vi "Get NART response from response string.vi"(0 "Expected Response":T1, 5 "Response Subtype":T2, 7 "Expected Message start (\"\":any)":string, 9 "TCP Line":string, 11 "error in (no error)":errorcluster) -> (8 "NART Message":T3, 15 "error out":errorcluster)   [LabVIEW 2011, in "ART2 Test Panel.lvlib"]
uses:
  ART2 Test Panel.lvlib
  NART/Controls/NART Message.ctl
  NART/Controls/NART TCP Response Types.ctl
  NART/Controls/NART Response Subtype.ctl
  <vilib>/Utility/error.llb/whitespace.ctl
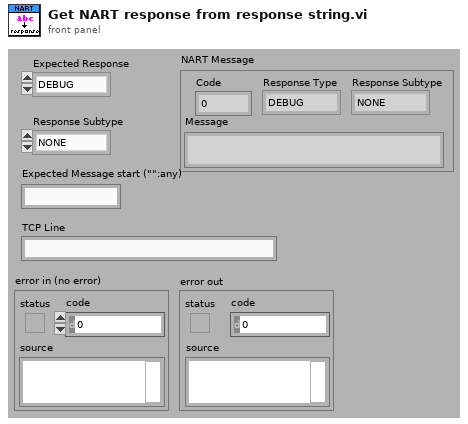
[diagram p1: front panel]
types:
  T1 = typedef "ART2 Test Panel.lvlib/NART TCP Response Types.ctl" = enum16{"DEBUG", "CONTROL", "INFO", "WARNING", "ERROR", "NONE"}
  T2 = typedef "ART2 Test Panel.lvlib/NART Response Subtype.ctl" = enum16{"NONE", "OK", "ON", "OFF", "BEGIN", "DONE"}
  T3 = typedef "ART2 Test Panel.lvlib/NART Message.ctl" = cluster{"Code":dbl, "Response Type":T1, "Response Subtype":T2, "Message":string}
  T4 = typedef "whitespace.ctl" = u16
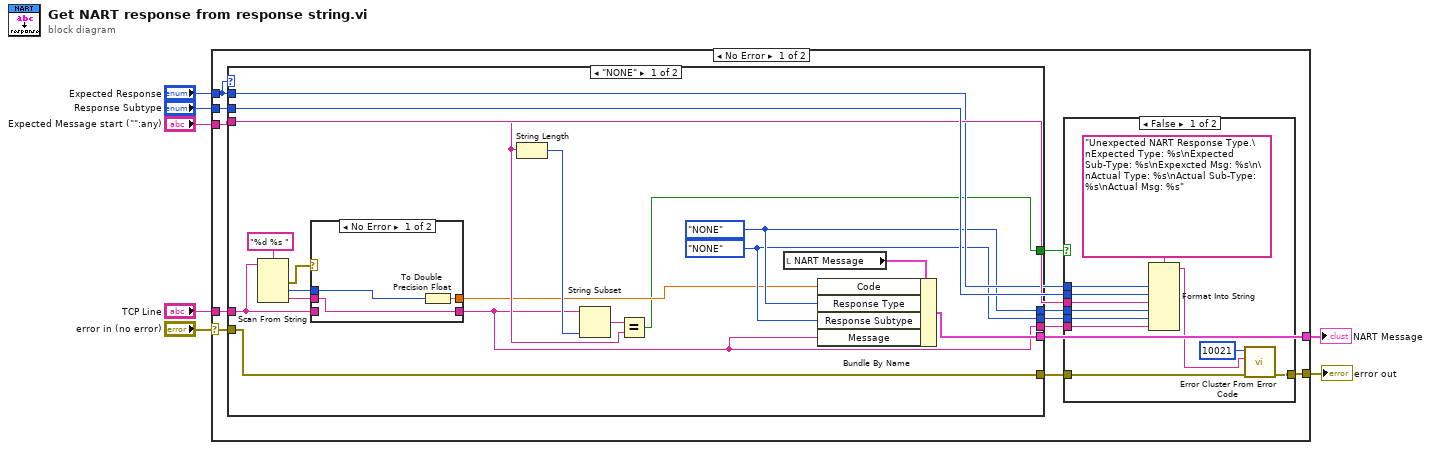
[diagram p0: block diagram]
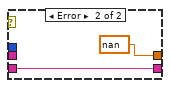
[diagram p2: hidden frame]
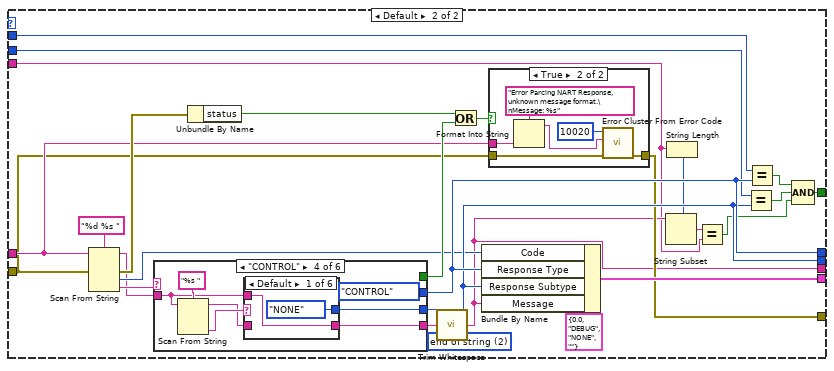
[diagram p3: hidden frame]
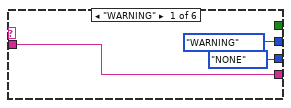
[diagram p5: hidden frame]
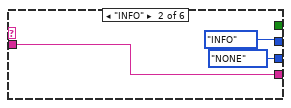
[diagram p6: hidden frame]
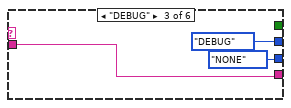
[diagram p7: hidden frame]
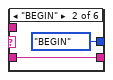
[diagram p8: hidden frame]
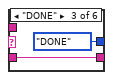
[diagram p9: hidden frame]
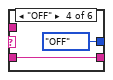
[diagram p10: hidden frame]
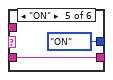
[diagram p11: hidden frame]
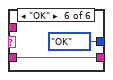
[diagram p12: hidden frame]
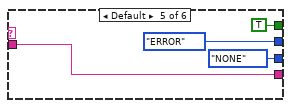
[diagram p13: hidden frame]
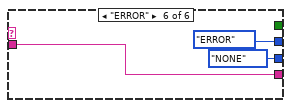
[diagram p14: hidden frame]
diagram:
  n1 = case shown="No Error" "error in (no error)" {
    selector: "error in (no error)" -> [w11 w122]
    tunnel: [w19 w122] -> w7
    tunnel: [w18 _] -> w6
    tunnel: "Response Subtype" -> [w15 _]
    tunnel: "Expected Response" -> [w8 _]
    tunnel: "TCP Line" -> [w12 _]
    tunnel: "Expected Message start (\"\":any)" -> [w9 _]
    frame No Error {
      n2 = case shown="\"NONE\"" w8 {
        tunnel: [w32 w67] -> w18
        tunnel: [w30 w66] -> w17
        tunnel: [w29 w65] -> w16
        tunnel: w15 -> [_ w64]
        tunnel: w8 -> [_ w63]
        tunnel: [w22 w62] -> w14
        tunnel: [w21 w51] -> w13
        tunnel: w12 -> [w20 w50]
        tunnel: w11 -> [w21 w49]
        tunnel: [w27 w43] -> w10
        tunnel: w9 -> [w34 w42]
        frame "NONE" {
          w29 = NART_Response_Subtype."NONE" ("Response Subtype")
          w30 = NART_TCP_Response_Types."NONE" ("Response Type")
          n3 = Scan From String(format string="%d %s ", input string=w20) -> (error out=w25:errorcluster, output 1=w24:i32, output 2=w23:string)  [unwired: 4 in, 2 out]
          n4 = case shown="No Error" w25 {
            tunnel: w20 -> [_ w40]
            tunnel: [w38 nan ("Code")] -> w28
            tunnel: [w36 w40] -> w27
            tunnel: w24 -> [w37 _]
            tunnel: w23 -> [w36 _]
            frame No Error {
              n5 = To Double Precision Float(number=w37) -> (double precision float=w38:dbl)
            }
            frame Error {
            }
          }
          n6 = String Length(string=w34) -> (length=w33:i32)
          n7 = String Subset(string=w27, length (rest)=w33) -> (substring=w35:string)  [unwired: 1 in]
          n8 = Equal?(x=w35, y=w34) -> (x = y?=w22:bool)
          n9 = local read "NART Message"() -> (w31:T3)
          n10 = Bundle By Name(cluster=w31, "Code"=w28, "Response Type"=w30, "Response Subtype"=w29, "Message"=w27) -> (w32:T3)
        }
        frame Default {
          w46 = T4 2 items=["both", "start of string", "end of string"] ("location (both)")
          n11 = Scan From String(format string="%d %s ", input string=w50, error in=w49) -> (remaining string=w48:string, error out=w56:errorcluster, output 1=w55:i32, output 2=w57:string)  [unwired: 3 in, 1 out]
          n12 = case shown="\"CONTROL\"" w57 {
            tunnel: [_ _ _ _ TRUE _] -> w59
            tunnel: [NART_TCP_Response_Types."WARNING" ("Response Type") NART_TCP_Response_Types."INFO" ("Response Type") NART_TCP_Response_Types."DEBUG" ("Response Type") NART_TCP_Response_Types."CONTROL" ("Response Type") NART_TCP_Response_Types."ERROR" ("Response Type") NART_TCP_Response_Types."ERROR" ("Response Type")] -> w66
            tunnel: w48 -> [w76 w79 w82 w87 w104 w108]
            tunnel: [w76 w79 w82 w86 w104 w108] -> w47
            tunnel: [NART_Response_Subtype."NONE" ("Response Subtype") NART_Response_Subtype."NONE" ("Response Subtype") NART_Response_Subtype."NONE" ("Response Subtype") w85 NART_Response_Subtype."NONE" ("Response Subtype") NART_Response_Subtype."NONE" ("Response Subtype")] -> w65
            frame "WARNING" {
            }
            frame "INFO" {
            }
            frame "DEBUG" {
            }
            frame "CONTROL" {
              n13 = Scan From String(format string="%s ", input string=w87) -> (remaining string=w84:string, output 1=w88:string)  [unwired: 3 in, 2 out]
              n14 = case shown="Default" w88 {
                tunnel: w84 -> [_ w93 w95 w97 w99 w101]
                tunnel: w87 -> [w92 _ _ _ _ _]
                tunnel: [w92 w93 w95 w97 w99 w101] -> w86
                tunnel: [NART_Response_Subtype."NONE" ("Response Subtype") NART_Response_Subtype."BEGIN" ("Response Subtype") NART_Response_Subtype."DONE" ("Response Subtype") NART_Response_Subtype."OFF" ("Response Subtype") NART_Response_Subtype."ON" ("Response Subtype") NART_Response_Subtype."OK" ("Response Subtype")] -> w85
                frame Default {
                }
                frame "BEGIN" {
                }
                frame "DONE" {
                }
                frame "OFF" {
                }
                frame "ON" {
                }
                frame "OK" {
                }
              }
            }
            frame Default {
            }
            frame "ERROR" {
            }
          }
          n15 = Unbundle By Name(w56) -> ("status"=w58:bool)
          n16 = call <vilib>:"Trim Whitespace.vi"("string"=w47, "location (both)"=w46) -> ("trimmed string"=w43:string)
          n17 = Or(x=w58, y=w59) -> (x .or. y?=w52:bool)
          n18 = Bundle By Name(cluster=T3 {"Code"=0.0, "Response Type"=enum."DEBUG", "Response Subtype"=enum."NONE", "Message"=""} ("NART Message"), "Code"=w55, "Response Type"=w66, "Response Subtype"=w65, "Message"=w43) -> (w67:T3)
          n19 = case shown="True" w52 {
            tunnel: [w68 w71] -> w51
            tunnel: w50 -> [_ w70]
            tunnel: w49 -> [w68 w69]
            frame False {
            }
            frame True {
              n20 = Format Into String(format string="Error Parcing NART Response, unknown message format.\nMessage: %s", w70) -> (resulting string=w74:string)  [unwired: 2 in, 1 out]
              n21 = call <vilib>:"Error Cluster From Error Code.vi"("error in (no error)"=w69, "error message (\"\")"=w74, "error code (0)"=10020) -> ("error out"=w71:errorcluster)  [unwired: 6 in]
            }
          }
          n22 = String Length(string=w42) -> (length=w45:i32)
          n23 = String Subset(string=w43, length (rest)=w45) -> (substring=w44:string)  [unwired: 1 in]
          n24 = Equal?(x=w44, y=w42) -> (x = y?=w41:bool)
          n25 = Equal?(x=w64, y=w65) -> (x = y?=w61:bool)
          n26 = Equal?(x=w63, y=w66) -> (x = y?=w60:bool)
          n27 = Compound Arithmetic op=AND(w60, w61, w41) -> (w62:bool)
        }
      }
      n28 = case shown="False" w14 {
        tunnel: w13 -> [w120 w121]
        tunnel: [w112 w121] -> w19
        tunnel: w8 -> [w116 _]
        tunnel: w15 -> [w115 _]
        tunnel: w16 -> [w114 _]
        tunnel: w17 -> [w113 _]
        tunnel: w9 -> [w111 _]
        tunnel: w10 -> [w110 _]
        frame False {
          n29 = Format Into String(format string="Unexpected NART Response Type.\nExpected Type: %s\nExpected Sub-Type: %s\nExpexcted Msg: %s\n\nActual Type: %s\nActual Sub-Type: %s\nActual Msg: %s", w116, w115, w111, w113, w114, w110) -> (resulting string=w117:string)  [unwired: 2 in, 1 out]
          n30 = call <vilib>:"Error Cluster From Error Code.vi"("error in (no error)"=w120, "error message (\"\")"=w117, "error code (0)"=10021) -> ("error out"=w112:errorcluster)  [unwired: 6 in]
        }
        frame True {
        }
      }
    }
    frame Error {
    }
  }
  "error out" <- w7
  "NART Message" <- w6
